vi "Close.vi"(8 "Error In":errorcluster, 11 "Dashboard":refnum<class "Dashboard.lvclass">) -> (0 "Error Out":errorcluster)   [LabVIEW 2019, in "Dashboard.lvclass"]
uses:
  Dashboard.lvclass
  <vilib>/FPGAPlugInAG/Dynamic/niLvFpga_Close_Dynamic.vi
  <vilib>/rvi/interface/nirviCloseFPGA/nirviCloseFPGA.xnode
  Controls/FPGA Reference.ctl
  <vilib>/Memosfet/OpenWeatherAPI/Open Weather Session/Open Weather Session.lvclass
  Display Manager/Display Manager.lvclass
  Audio Analyzer/Audio Analyzer.lvclass
  Draw Frame/Draw Frame.lvclass
  Error Handling/Error Handling.lvclass
  Sequencer/Sequencer.lvclass
  <vilib>/Memosfet/myRIO-Neopixel/RT/Display/Display.lvclass
  Central Message Handler/Central Message Handler.lvclass
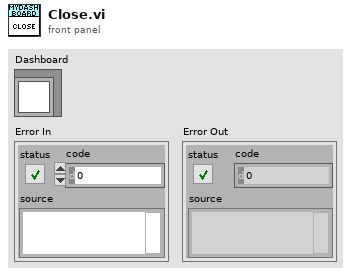
[diagram p1: front panel]
types:
  T1 = typedef "Dashboard.lvclass/Data.ctl" = cluster{"Central Message Handler":refnum<class "Central Message Handler.lvclass">, "Display":refnum<class "Display.lvclass">, "FPGA Reference":T2, "Open Weather Session":refnum<class "Open Weather Session.lvclass">, "Processes":T3}
  T2 = typedef "Dashboard.lvclass/FPGA Reference.ctl" = refnum<k20>
  T3 = typedef "Dashboard.lvclass/Processes.ctl" = cluster{"Display Manager":refnum<class "Display Manager.lvclass">, "Audio Analyzer":refnum<class "Audio Analyzer.lvclass">, "Draw Frame":refnum<class "Draw Frame.lvclass">, "Error Handling":refnum<class "Error Handling.lvclass">, "Sequencer":refnum<class "Sequencer.lvclass">}
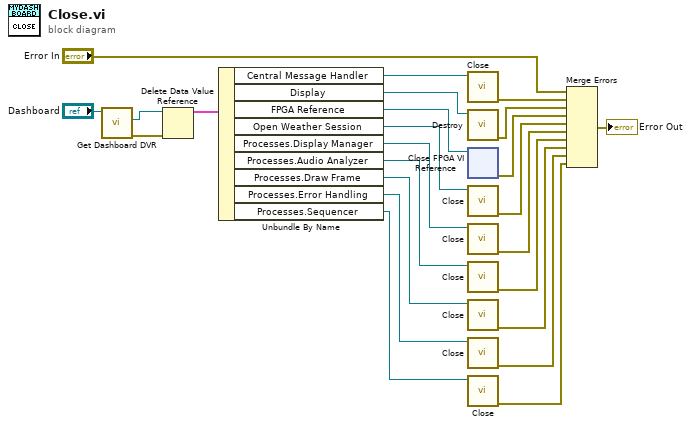
[diagram p0: block diagram]
diagram:
  n1 = call "Get Dashboard DVR.vi"("Dashboard In"="Dashboard") -> ("Error Out"=w22:errorcluster, "DVR"=w23:refnum<data-value>)  [unwired: 8 in, 1 out]
  n2 = Delete Data Value Reference(data value reference=w23, error in=w22) -> (data value=w21:T1)  [unwired: 1 out]
  n3 = Unbundle By Name(w21) -> ("Central Message Handler"=w18:refnum<class "Central Message Handler.lvclass">, "Display"=w17:refnum<class "Display.lvclass">, "FPGA Reference"=w20:T2, "Open Weather Session"=w19:refnum<class "Open Weather Session.lvclass">, "Processes.Display Manager"=w16:refnum<class "Display Manager.lvclass">, "Processes.Audio Analyzer"=w15:refnum<class "Audio Analyzer.lvclass">, "Processes.Draw Frame"=w14:refnum<class "Draw Frame.lvclass">, "Processes.Error Handling"=w13:refnum<class "Error Handling.lvclass">, "Processes.Sequencer"=w12:refnum<class "Sequencer.lvclass">)
  n4 = call "Close.vi"("Central Message Handler"=w18) -> ("Error Out"=w10:errorcluster)  [unwired: 10 in]
  n5 = call <vilib>:"Destroy.vi"("Display In"=w17) -> ("Error Out"=w9:errorcluster)  [unwired: 10 in]
  n6 = xnode "Close FPGA VI Reference"("FPGA VI Reference In"=w20) -> ("error out"=w8:errorcluster)  [unwired: 1 in]
  n7 = call-dynamic "Close.vi"("Open Weather Session In"=w19) -> ("Error Out"=w7:errorcluster)  [unwired: 10 in]
  n8 = call-dynamic "Close.vi"("Display Manager In"=w16) -> ("Error Out"=w6:errorcluster)  [unwired: 10 in]
  n9 = call-dynamic "Close.vi"("Audio Analyzer In"=w15) -> ("Error Out"=w5:errorcluster)  [unwired: 10 in]
  n10 = call-dynamic "Close.vi"("Draw Frame In"=w14) -> ("Error Out"=w4:errorcluster)  [unwired: 10 in]
  n11 = call-dynamic "Close.vi"("Error Handling In"=w13) -> ("Error Out"=w3:errorcluster)  [unwired: 10 in]
  n12 = call-dynamic "Close.vi"("Sequencer In"=w12) -> ("Error Out"=w2:errorcluster)  [unwired: 10 in]
  n13 = Merge Errors("Error In", w10, w9, w8, w7, w6, w5, w4, w3, w2) -> (→"Error Out":errorcluster)
